vi "漂移技术参数设置.vi"(11 "输入簇":T1) -> (3 "输出簇":T1)   [LabVIEW 2016, in "数据查询.lvlib"]
panel:
  in  "选项卡控件":enum32{"氨氮", "总磷", "总氮", "CODMn", "CODCr"}(tab)
  in  "技术要求":dbl format="%#_gmg/L"
  in  "24H漂移技术要求":dbl format="%#_g%"
  in  "技术要求2":dbl format="%#_g%"
  in  "24H漂移技术要求2":dbl format="%#_g%"
  in  "技术要求":dbl format="%#_gmg/L"
  in  "24H漂移技术要求":dbl format="%#_g%"
  in  "技术要求2":dbl format="%#_g%"
  in  "24H漂移技术要求2":dbl format="%#_g%"
  in  "技术要求":dbl format="%#_gmg/L"
  in  "24H漂移技术要求":dbl format="%#_g%"
  in  "技术要求2":dbl format="%#_g%"
  in  "24H漂移技术要求2":dbl format="%#_g%"
  in  "技术要求":dbl format="%#_gmg/L"
  in  "24H漂移技术要求":dbl format="%#_g%"
  in  "技术要求2":dbl format="%#_g%"
  in  "24H漂移技术要求2":dbl format="%#_g%"
  in  "技术要求":dbl format="%#_gmg/L"
  in  "24H漂移技术要求":dbl format="%#_g%"
  in  "技术要求2":dbl format="%#_g%"
  in  "24H漂移技术要求2":dbl format="%#_g%"
  # "漂移技术要求"
  # "零点核查"
  # "±"
  # "±"
  # "跨度核查"
  # "±"
  # "±"
  # "零点核查"
  # "±"
  # "±"
  # "跨度核查"
  # "±"
  # "±"
  # "零点核查"
  # "±"
  # "±"
  # "跨度核查"
  # "±"
  # "±"
  # "零点核查"
  # "±"
  # "±"
  # "跨度核查"
  # "±"
  # "±"
  # "零点核查"
  # "±"
  # "±"
  # "跨度核查"
  # "±"
  # "±"
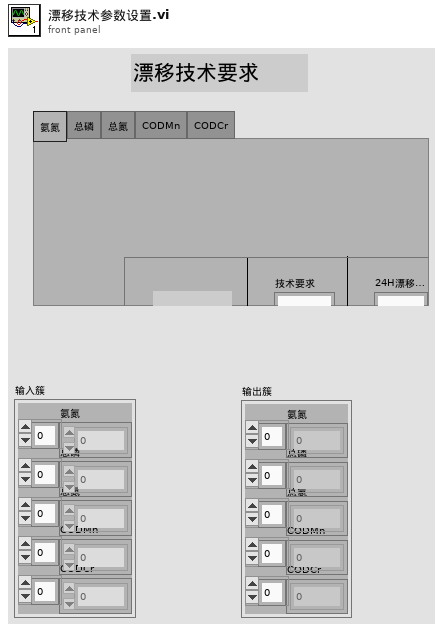
[diagram p1: front panel]
types:
  T1 = cluster{"氨氮":dbl[], "总磷":dbl[], "总氮":dbl[], "CODMn":dbl[], "CODCr":dbl[]}
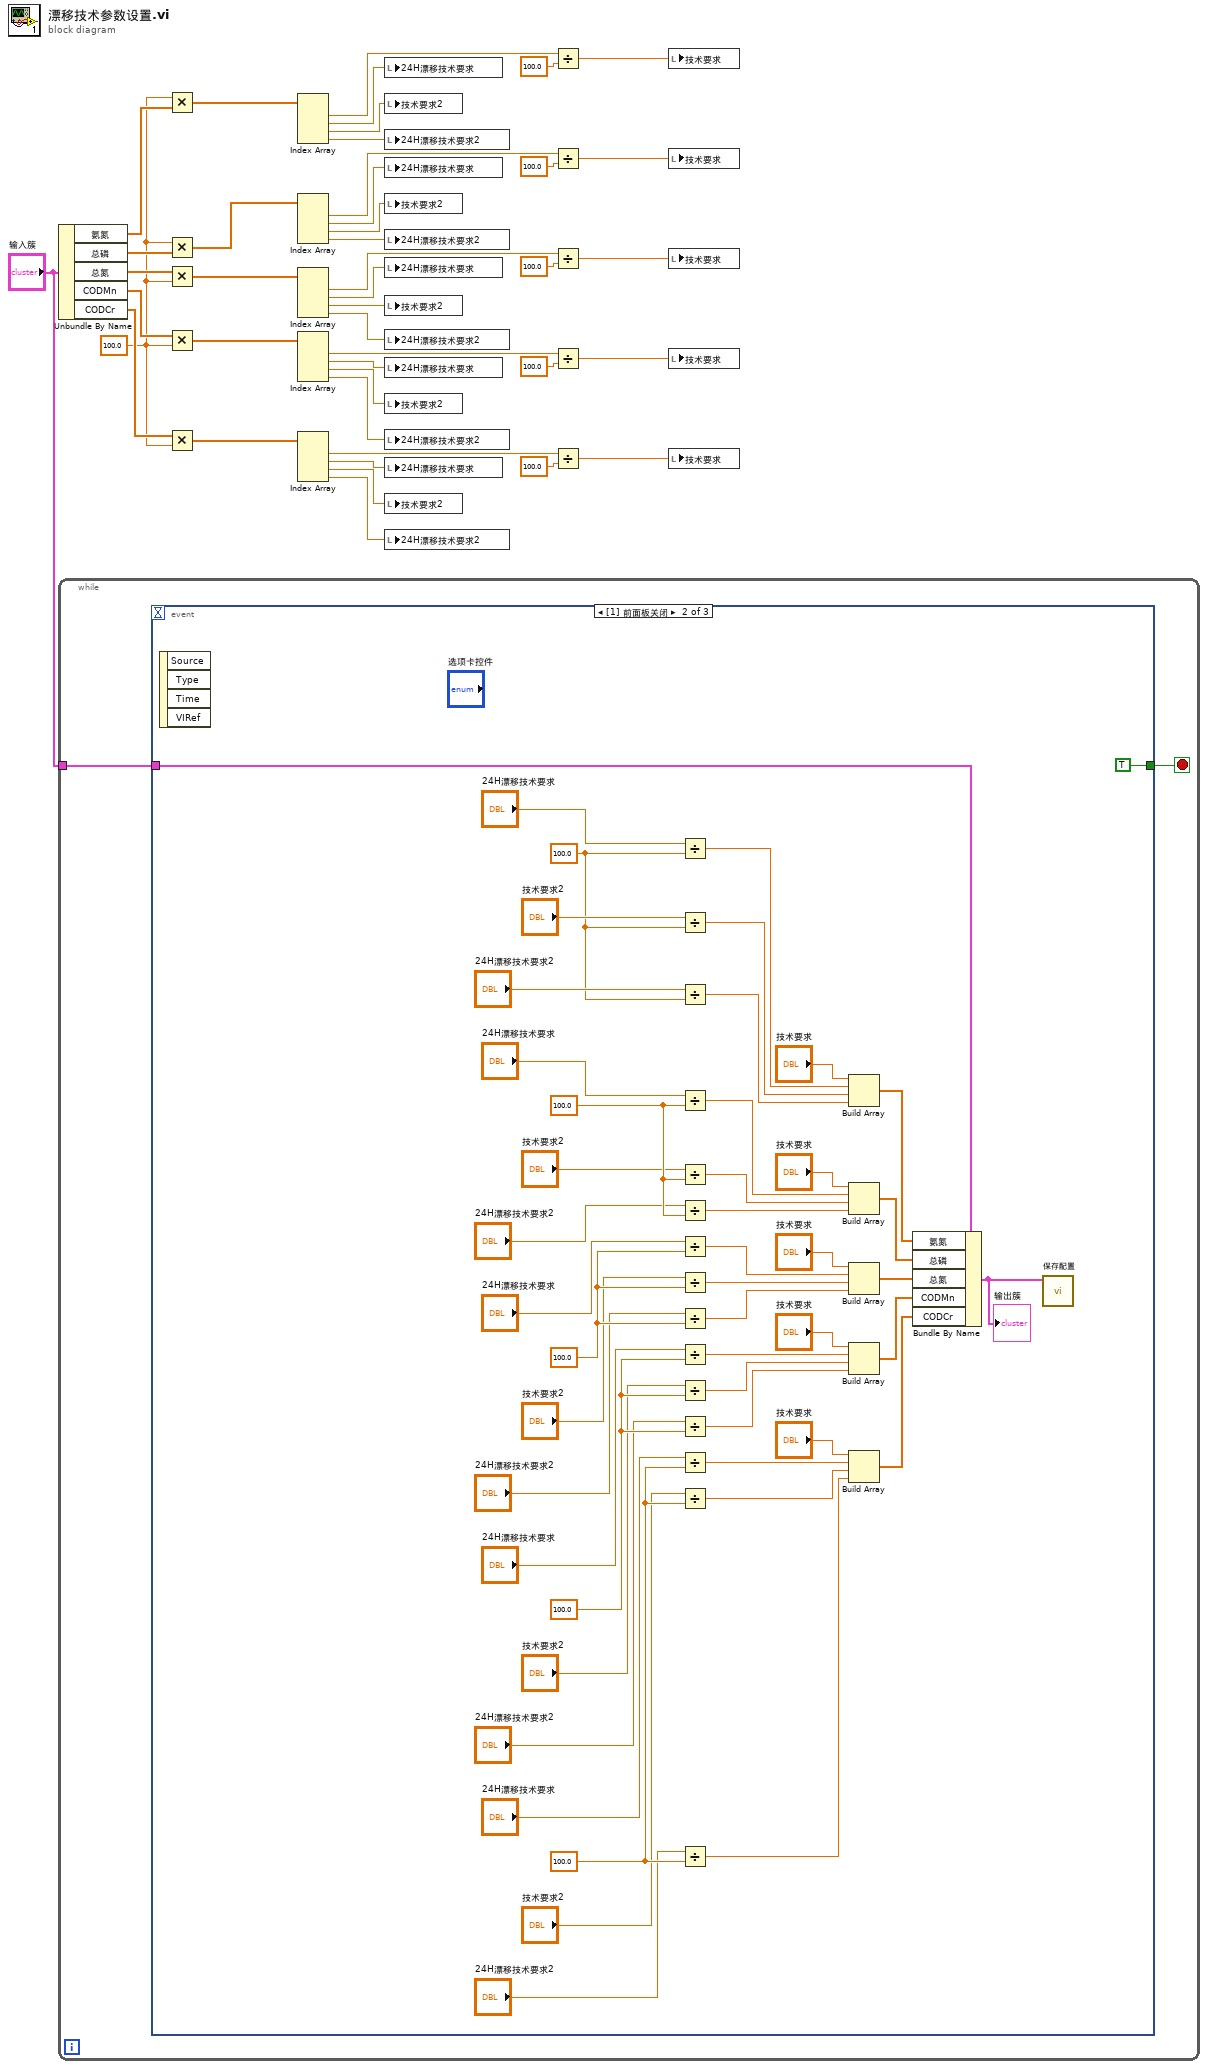
[diagram p0: block diagram]
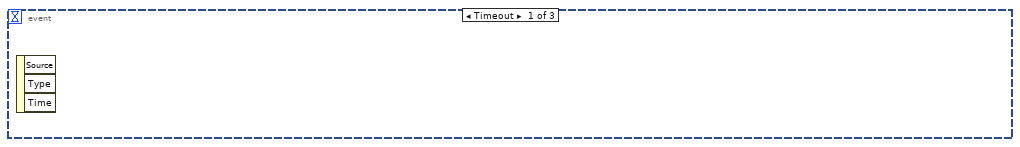
[diagram p2: hidden frame]
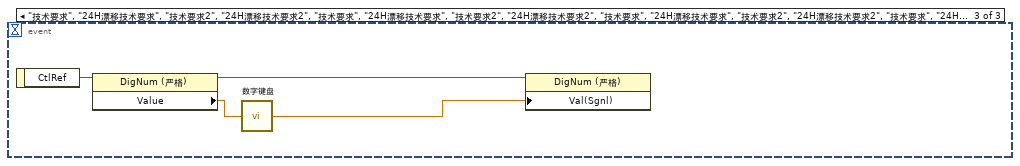
[diagram p3: hidden frame]
diagram:
  w17 = 100.0
  n1 = Unbundle By Name("输入簇") -> ("氨氮"=w42:dbl[], "总磷"=w38:dbl[], "总氮"=w37:dbl[], "CODMn"=w36:dbl[], "CODCr"=w35:dbl[])
  n2 = while {
    tunnel: "输入簇" -> [w43]
    stop <- w44 stop-if-true
    n3 = event shown="[1] 前面板关闭" {
      selector: _ -> [_ _ _]
      dyn-events: _ -> [_ _ _]
      timeout: _ -> [_ _ _]
      tunnel: [_ TRUE _] -> w44
      tunnel: w43 -> [_ w45 _]
      event Timeout {
        n4 = event-data() -> ()  [unwired: 1 in, 3 out]
      }
      event Panel Close {
        w55 = 100.0 ("x")
        w64 = 100.0 ("x")
        w73 = 100.0 ("x")
        w83 = 100.0 ("x")
        w84 = 100.0 ("x")
        n5 = event-data() -> ()  [unwired: 1 in, 4 out]
        n6 = Divide(x="24H漂移技术要求", y=w84) -> (x/y=w89:dbl)
        n7 = Divide(x="技术要求2", y=w84) -> (x/y=w90:dbl)
        n8 = Divide(x="24H漂移技术要求2", y=w84) -> (x/y=w91:dbl)
        n9 = Divide(x="24H漂移技术要求", y=w83) -> (x/y=w79:dbl)
        n10 = Divide(x="技术要求2", y=w83) -> (x/y=w75:dbl)
        n11 = Divide(x="24H漂移技术要求2", y=w83) -> (x/y=w74:dbl)
        n12 = Divide(x="24H漂移技术要求", y=w73) -> (x/y=w72:dbl)
        n13 = Divide(x="技术要求2", y=w73) -> (x/y=w71:dbl)
        n14 = Divide(x="24H漂移技术要求2", y=w73) -> (x/y=w70:dbl)
        n15 = Divide(x="24H漂移技术要求", y=w64) -> (x/y=w63:dbl)
        n16 = Divide(x="技术要求2", y=w64) -> (x/y=w62:dbl)
        n17 = Divide(x="24H漂移技术要求2", y=w64) -> (x/y=w61:dbl)
        n18 = Divide(x="24H漂移技术要求", y=w55) -> (x/y=w54:dbl)
        n19 = Divide(x="技术要求2", y=w55) -> (x/y=w53:dbl)
        n20 = Divide(x="24H漂移技术要求2", y=w55) -> (x/y=w52:dbl)
        n21 = Build Array("技术要求", w89, w90, w91) -> (w82:dbl[])
        n22 = Build Array("技术要求", w79, w75, w74) -> (w81:dbl[])
        n23 = Build Array("技术要求", w72, w71, w70) -> (w65:dbl[])
        n24 = Build Array("技术要求", w63, w62, w61) -> (w56:dbl[])
        n25 = Build Array("技术要求", w54, w53, w52) -> (w47:dbl[])
        n26 = Bundle By Name(cluster=w45, "氨氮"=w82, "总磷"=w81, "总氮"=w65, "CODMn"=w56, "CODCr"=w47) -> (w46:T1)
        "输出簇" <- w46
        n27 = call "保存配置.vi"("输入簇"=w46) -> ()  [unwired: 11 in]
      }
      event "技术要求", "24H漂移技术要求", "技术要求2", "24H漂移技术要求2", "技术要求", "24H漂移技术要求", "技术要求2", "24H漂移技术要求2", "技术要求", "24H漂移技术要求", "技术要求2", "24H漂移技术要求2", "技术要求", "24H漂移技术要求", "技术要求2", "24H漂移技术要求2", "技术要求", "24H漂移技术要求", "技术要求2", "24H漂移技术要求2": Mouse Down {
        n28 = event-data() -> ("CtlRef"=w96:refnum<vi>)  [unwired: 1 in]
        n29 = property class="DigNum (严格)"(reference=w96) -> (reference out=w94:refnum<vi>, "Value"=w95:dbl)  [unwired: 1 in, 1 out]
        n30 = call "数字键盘.vi"("OldNumber"=w95) -> ("NewNumber"=w93:sgl)
        n31 = property class="DigNum (严格)"(reference=w94, "Val(Sgnl)"=w93) -> ()  [unwired: 1 in, 2 out]
      }
    }
  }
  n32 = Multiply(x=w17, y=w42) -> (x*y=w22:dbl[])
  n33 = Multiply(x=w17, y=w38) -> (x*y=w21:dbl[])
  n34 = Multiply(x=w37, y=w17) -> (x*y=w20:dbl[])
  n35 = Multiply(x=w36, y=w17) -> (x*y=w19:dbl[])
  n36 = Multiply(x=w35, y=w17) -> (x*y=w18:dbl[])
  n37 = Index Array(array=w22) -> (element #1=w15:dbl, element #2=w41:dbl, element #3=w40:dbl, element #4=w39:dbl)  [unwired: 4 in]
  n38 = Index Array(array=w21) -> (element #1=w12:dbl, element #2=w34:dbl, element #3=w33:dbl, element #4=w32:dbl)  [unwired: 4 in]
  n39 = Index Array(array=w20) -> (element #1=w9:dbl, element #2=w31:dbl, element #3=w30:dbl, element #4=w29:dbl)  [unwired: 4 in]
  n40 = Index Array(array=w19) -> (element #1=w3:dbl, element #2=w28:dbl, element #3=w27:dbl, element #4=w26:dbl)  [unwired: 4 in]
  n41 = Index Array(array=w18) -> (element #1=w5:dbl, element #2=w25:dbl, element #3=w24:dbl, element #4=w23:dbl)  [unwired: 4 in]
  n42 = local write "24H漂移技术要求"(w41) -> ()
  n43 = local write "技术要求2"(w40) -> ()
  n44 = local write "24H漂移技术要求2"(w39) -> ()
  n45 = local write "24H漂移技术要求"(w34) -> ()
  n46 = local write "技术要求2"(w33) -> ()
  n47 = local write "24H漂移技术要求2"(w32) -> ()
  n48 = local write "24H漂移技术要求"(w31) -> ()
  n49 = local write "技术要求2"(w30) -> ()
  n50 = local write "24H漂移技术要求2"(w29) -> ()
  n51 = local write "24H漂移技术要求"(w28) -> ()
  n52 = local write "技术要求2"(w27) -> ()
  n53 = local write "24H漂移技术要求2"(w26) -> ()
  n54 = local write "24H漂移技术要求"(w25) -> ()
  n55 = local write "技术要求2"(w24) -> ()
  n56 = local write "24H漂移技术要求2"(w23) -> ()
  n57 = Divide(x=w15, y=100.0) -> (x/y=w16:dbl)
  n58 = Divide(x=w12, y=100.0) -> (x/y=w11:dbl)
  n59 = Divide(x=w9, y=100.0) -> (x/y=w8:dbl)
  n60 = Divide(x=w3, y=100.0) -> (x/y=w2:dbl)
  n61 = Divide(x=w5, y=100.0) -> (x/y=w4:dbl)
  n62 = local write "技术要求"(w16) -> ()
  n63 = local write "技术要求"(w11) -> ()
  n64 = local write "技术要求"(w8) -> ()
  n65 = local write "技术要求"(w2) -> ()
  n66 = local write "技术要求"(w4) -> ()
